vi "auto_alignment-v3-1.vi"(0 "meter-visa":refnum<visa-resource-name>, 1 "xStart":dbl=264.0 format="%#_13g", 2 "yStart":dbl=123.0 format="%#_13g", 3 "NM-params":T2={"alpha"=1.0, "gamma"=2.0, "rho"=0.5, "sigma"=0.5, "simplex L"=0.5}, 5 "PD Values":cluster{"PD1":dbl, "PD2":dbl, "PD3":dbl}, 7 "stage-refs":T1, 8 "NM-pts-tested":refnum<vi>, 9 "meter-error":errorcluster, 11 "stage-error":errorcluster, 12 "bar-note":u8, 13 "meas#":dbl format="%#_13g") -> (4 "Optimized Location":dbl[](array[numeric]), 6 "logfile-line-out":string, 10 "meter-error-out":errorcluster, 14 "run time (s)":dbl, 15 "stage-error-out":errorcluster)   [LabVIEW 2024]
uses:
  C:/Users/hpDIRC/Desktop/eic_dirc_daq-LabVIEW_new/Thorlabs.MotionControl.IntegratedStepperMotorsCLI.dll
  Thorlabs.MotionControl.IntegratedStepperMotorsCLI.dll
  C:/Users/hpDIRC/Desktop/eic_dirc_daq-LabVIEW_new/Thorlabs.MotionControl.Benchtop.StepperMotorCLI.dll
  Thorlabs.MotionControl.Benchtop.StepperMotorCLI.dll
  5b59031f-b1ff-41af-80a7-e72a33ebffa1.vi
  <vilib>/Analysis/baseanly.llb/Real Dot Product.vi
  <vilib>/Array/Sort 2D Array - Pop Stack.vi
  <vilib>/Array/Sort 2D Array - Push Stack.vi
  5b59031f-b1ff-41af-80a7-e72a33ebffa1.vi/269d4b3b-47f5-49e3-8884-44851e4dd9d5.vi
  5b59031f-b1ff-41af-80a7-e72a33ebffa1.vi/6d99389c-673d-4efb-bf33-19b32bcf4cf8.vi
  <vilib>/Analysis/NI_AALBase.lvlib
  <vilib>/Analysis/NI_AALPro.lvlib
panel:
  in  "fpga-ref-in":refnum<k20>
  out "z-angle converge":bool
  in  "z-angle-limit":dbl=0.04 caption="Z-Angle Convergence Goal"
  in  "squError-limit":dbl=0.04 caption="Squared Error Convergence Goal"
  out "angle-to-z":dbl
  out "squared error limit":bool
  out "SquError":dbl
  out "x_c":dbl[](array[numeric])
  out "x_e":dbl[](array[numeric])
  out "x_r":dbl[](array[numeric])
  out "x_o":dbl[](array[numeric])
  out "termination-test-simplex":dbl[][](array[numeric])
  out "timeout":bool
  out "simplex converge":bool
  out "value converge":bool
  out "simplex leg lengths":dbl[](array[numeric])
  out "std dev of simplex values":dbl
  out "nPts tested":dbl
  in  "simplex-limit":dbl=1e-06 caption="Simplex Length Convergence Goal" format="%#_13g"
  in  "value-limit":dbl=1e-06 caption="Value Convergence Goal" format="%#_13g"
  out "Pts Tested":dbl[][](array[numeric])
  in  "stop":bool
  # "Test Sub-Points"
  # "centroid"
  # "reflection point"
  # "expansion point"
  # "contraction point"
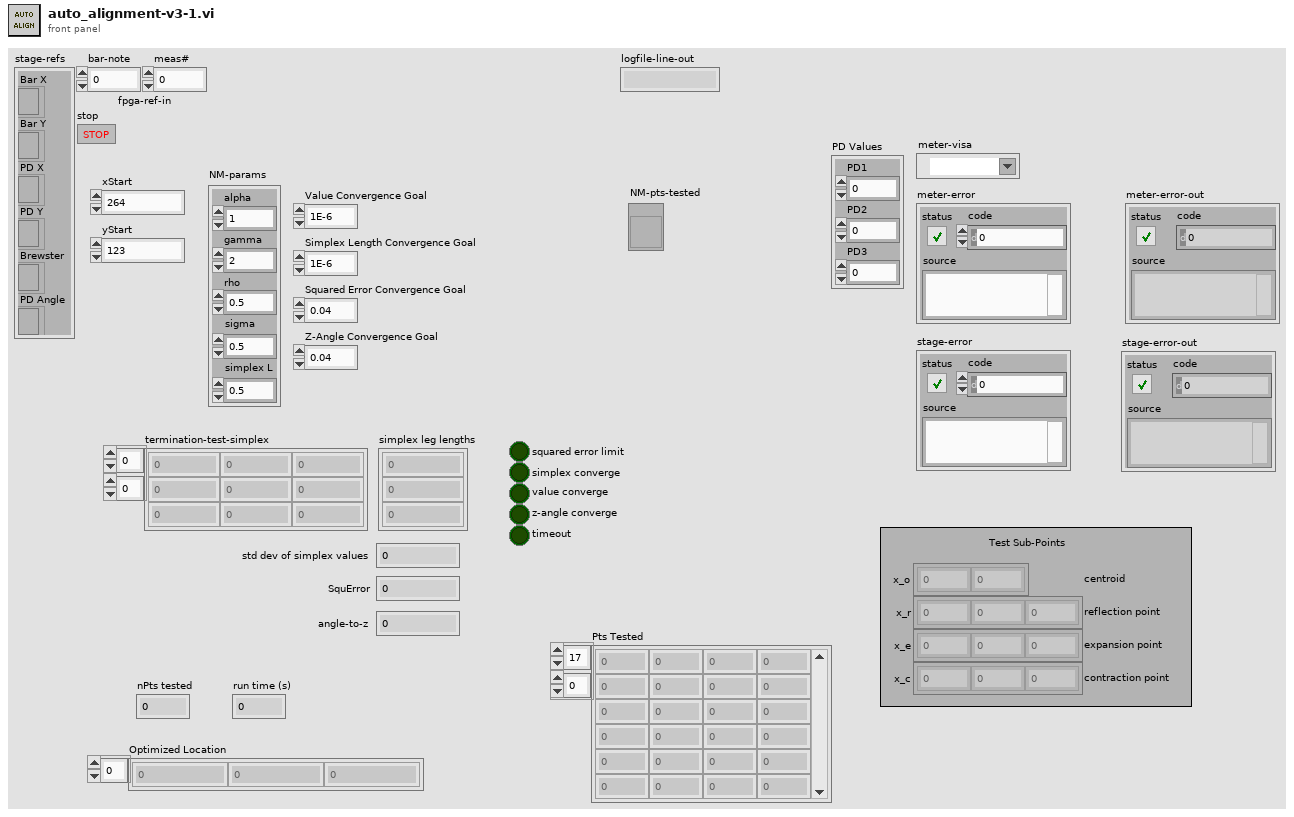
[diagram p1: front panel]
types:
  T1 = cluster{"Bar X":refnum<k24>, "Bar Y":refnum<k24>, "PD X":refnum<k24>, "PD Y":refnum<k24>, "Brewster":refnum<k24>, "PD Angle":refnum<k24>}
  T2 = cluster{"alpha":dbl, "gamma":dbl, "rho":dbl, "sigma":dbl, "simplex L":dbl}
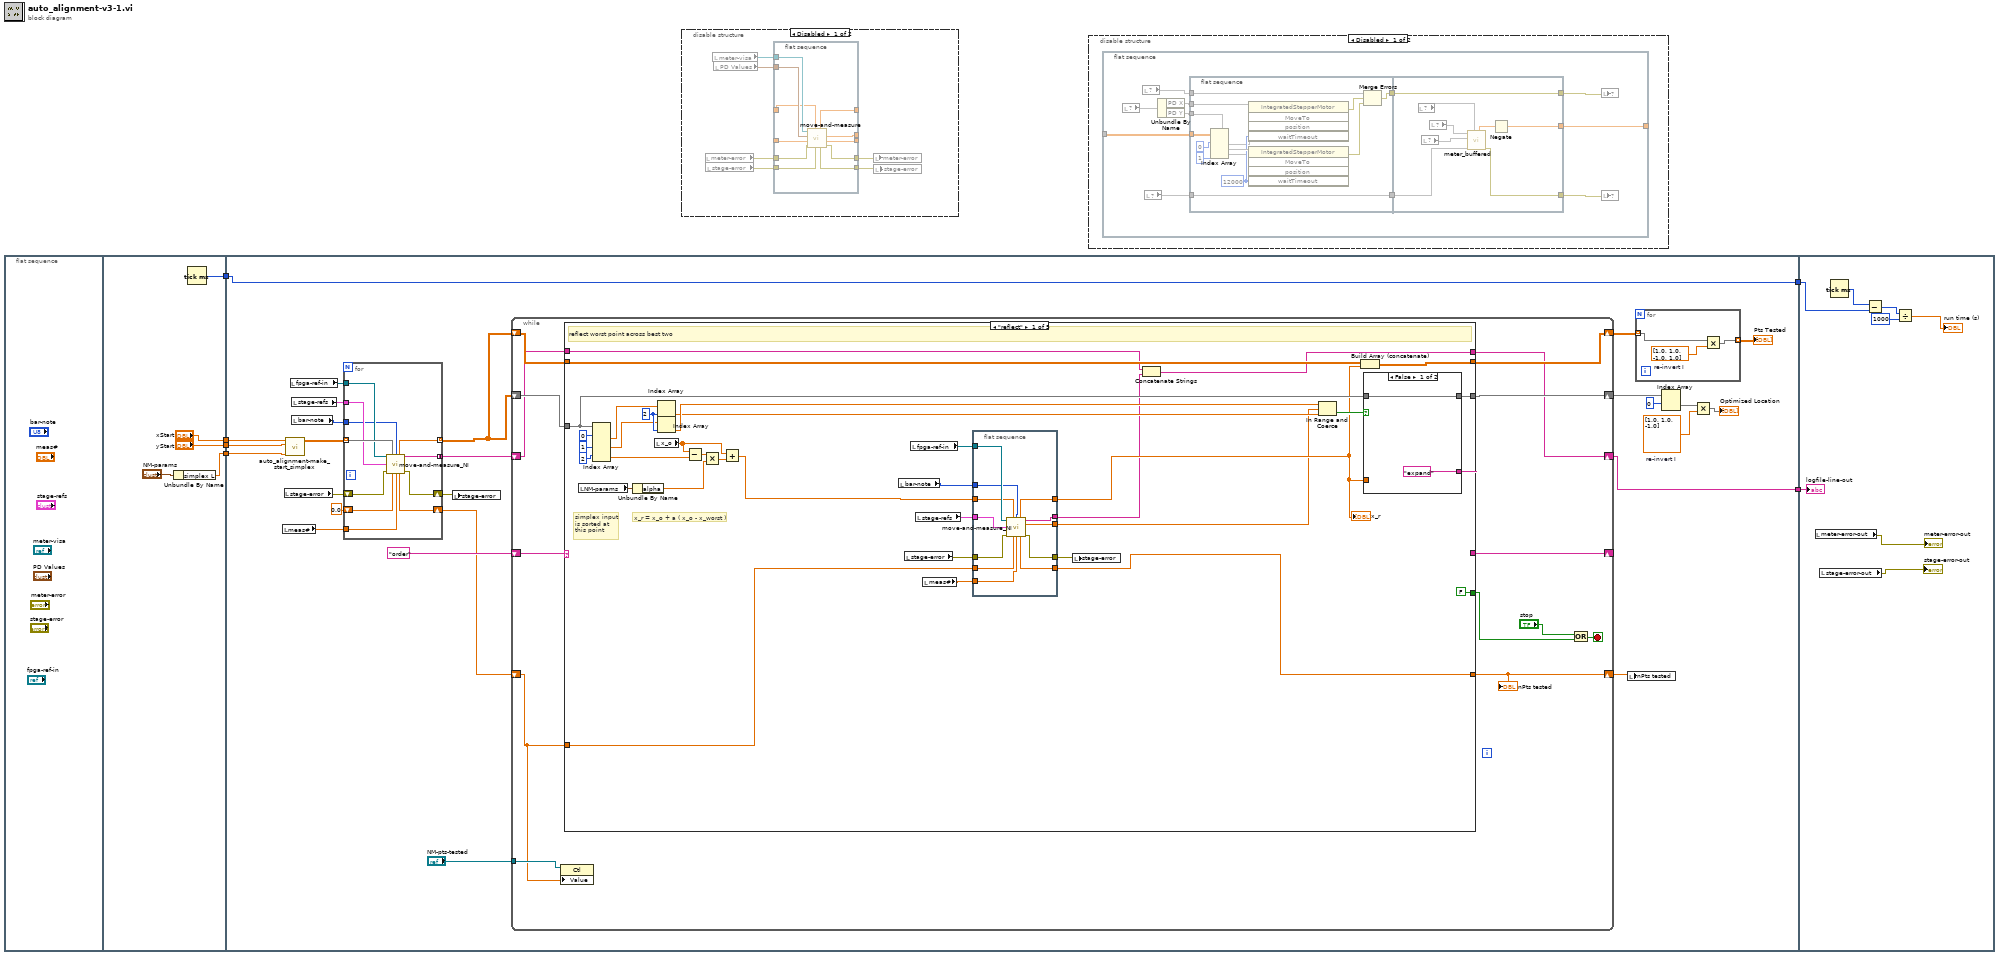
[diagram p0: block diagram]
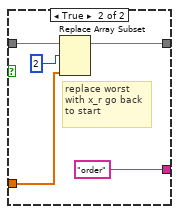
[diagram p4: hidden frame]
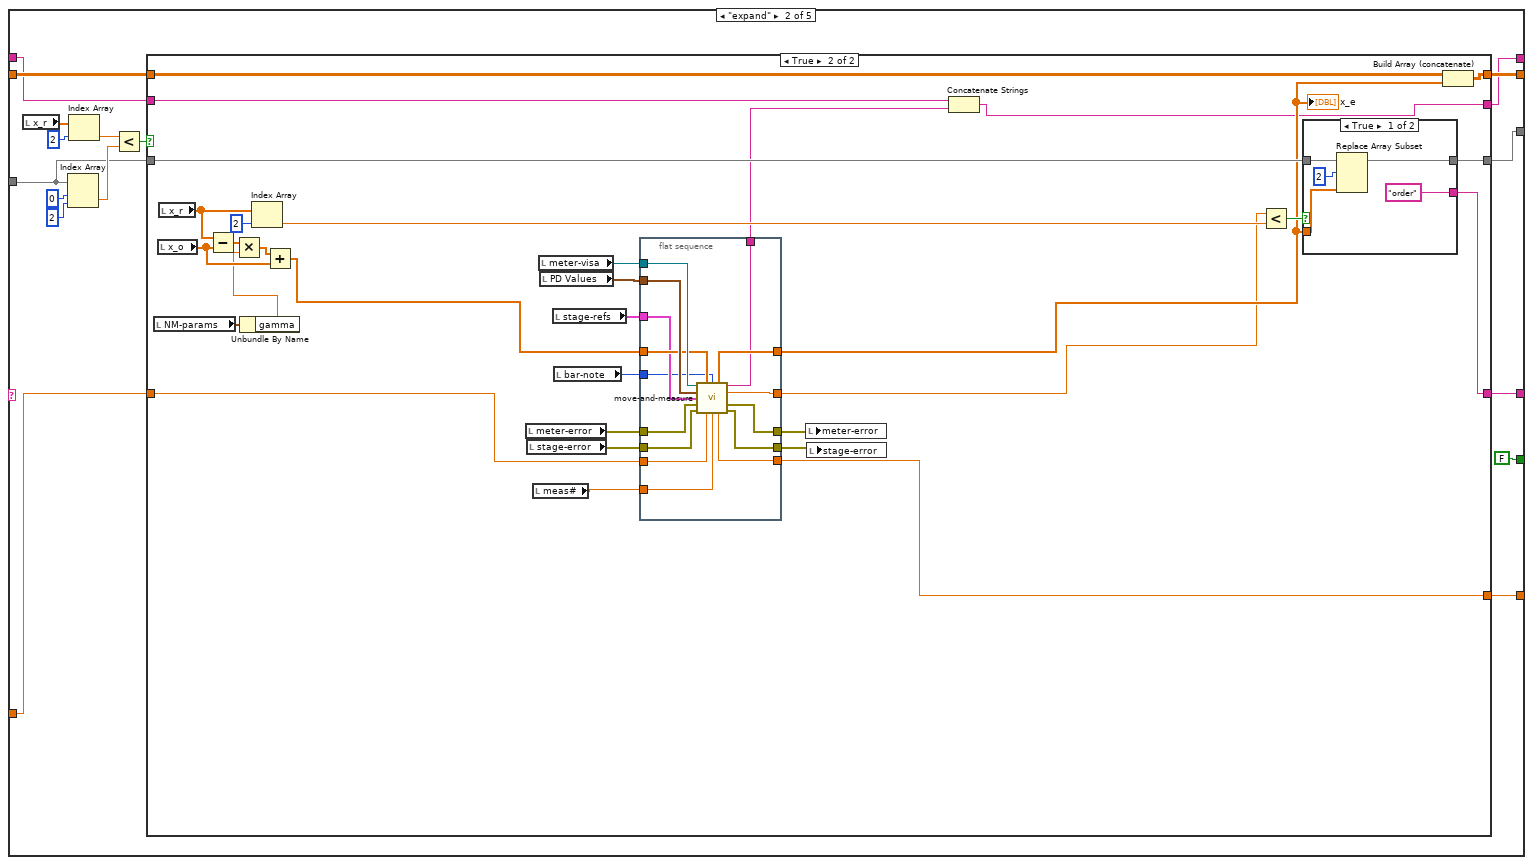
[diagram p5: hidden frame]
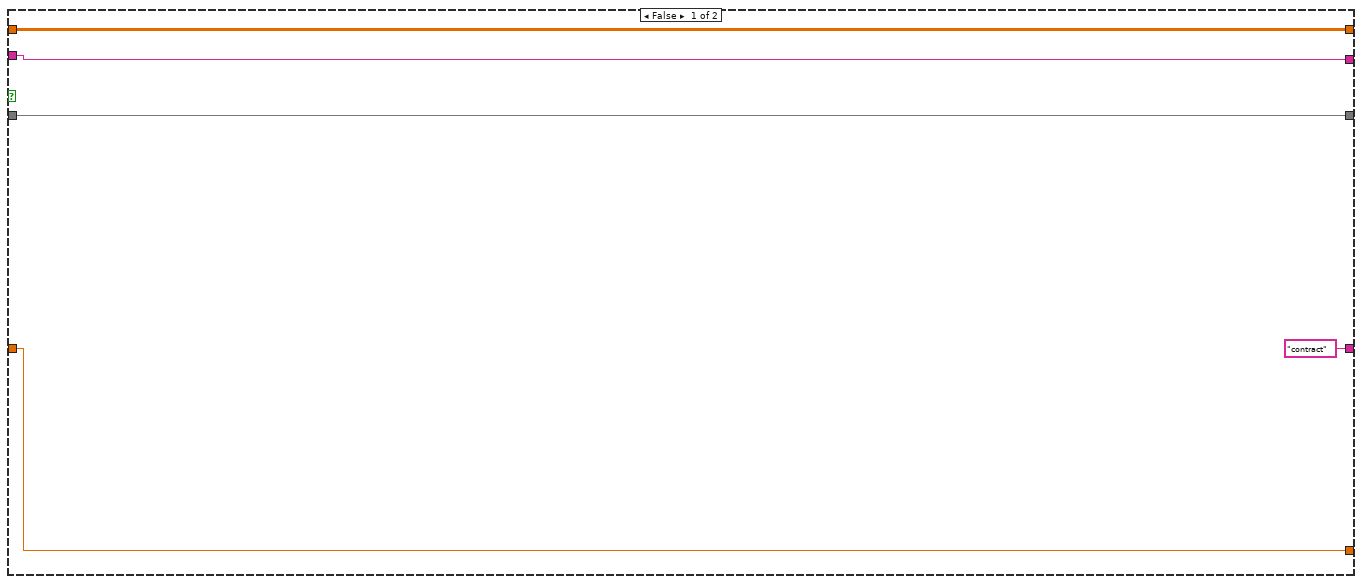
[diagram p6: hidden frame]
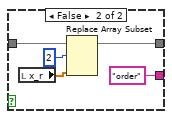
[diagram p7: hidden frame]
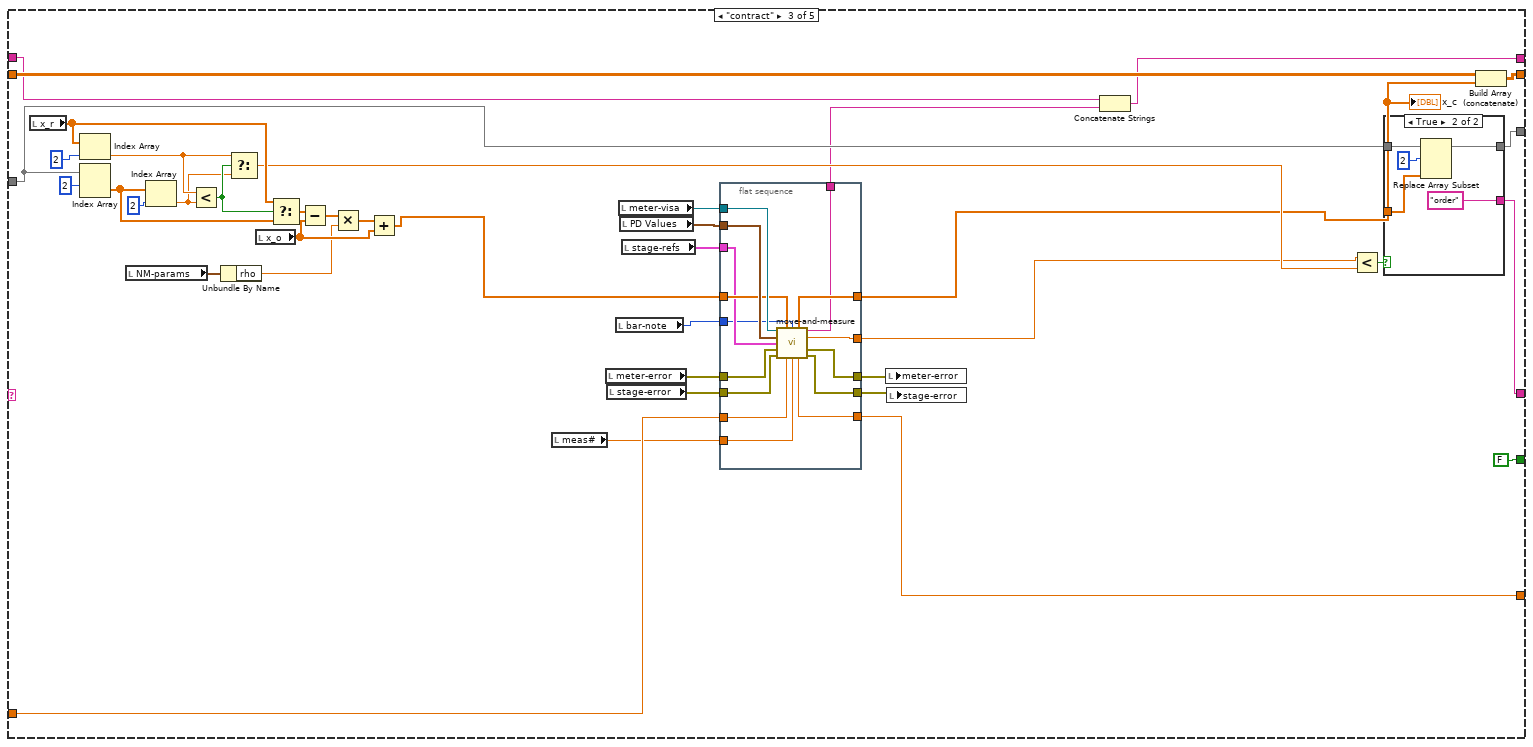
[diagram p8: hidden frame]
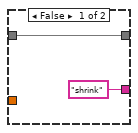
[diagram p9: hidden frame]
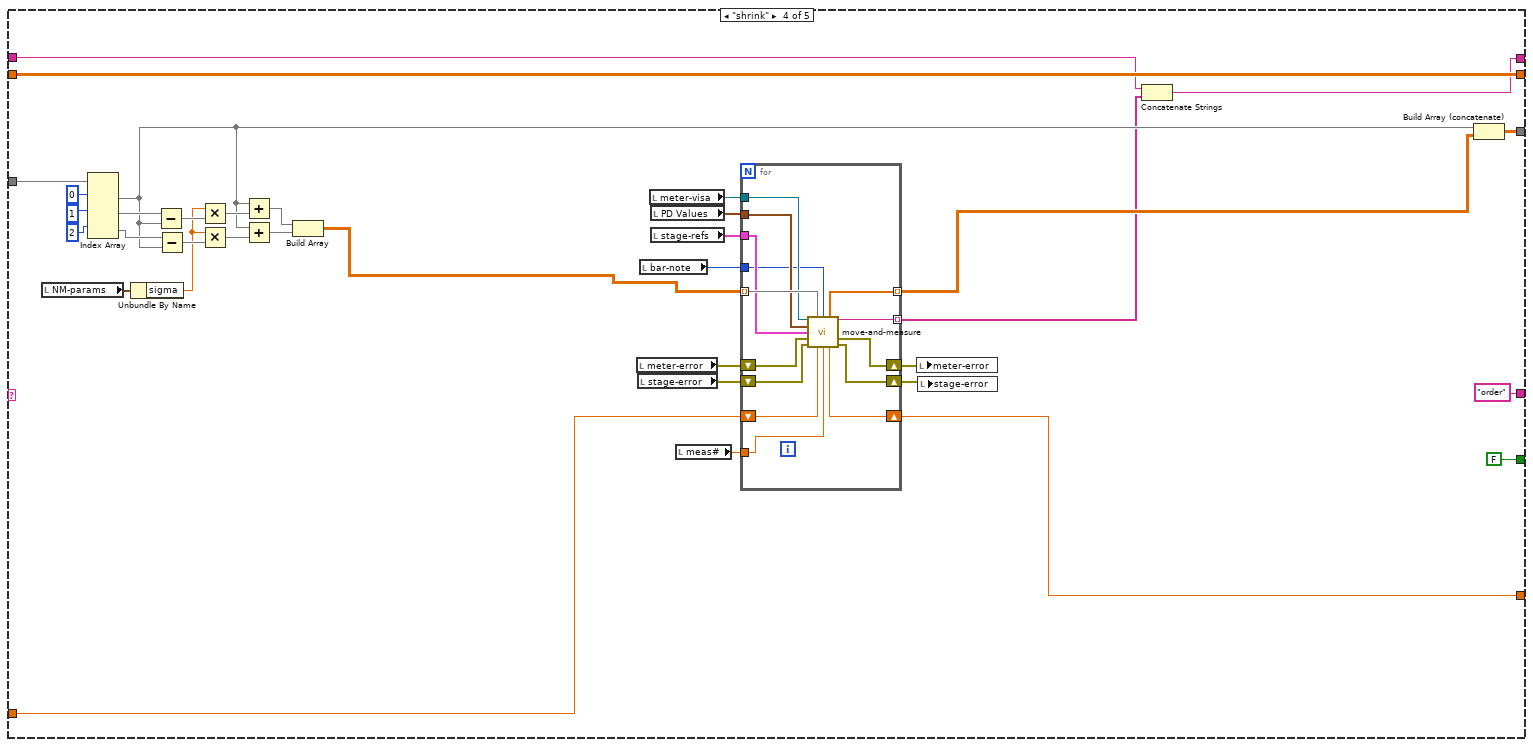
[diagram p10: hidden frame]
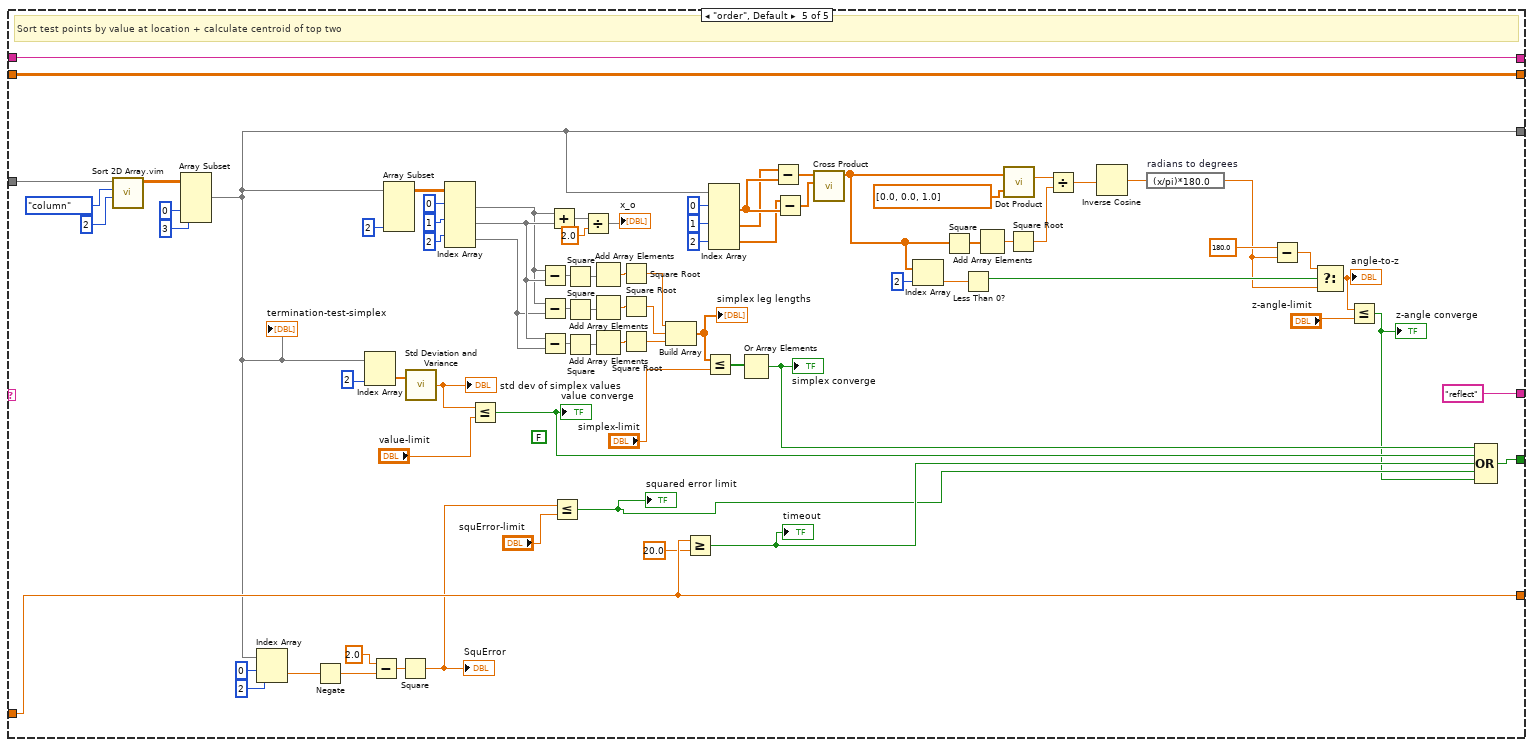
[diagram p11: hidden frame]
diagram:
  n1 = flat-sequence {
    tunnel: [w11] -> w6
    tunnel: ["yStart"] -> w4
    tunnel: ["xStart"] -> w3
    tunnel: [w9] -> w2
    tunnel: w6 -> [w36]
    tunnel: [w36] -> w5
    tunnel: w4 -> [w26]
    tunnel: w3 -> [w27]
    tunnel: w2 -> [w25]
    tunnel: [w15] -> w1
    tunnel: w5 -> [w394]
    tunnel: w1 -> [w388]
    frame #0 {
    }
    frame #1 {
      n2 = Unbundle By Name("NM-params") -> ("simplex L"=w9:dbl)
      n3 = Tick Count (ms)() -> (millisecond timer value=w11:u32)
    }
    frame #2 {
      w31 = dbl[] [1.0, 1.0, -1.0]  # re-invert I
      n4 = local read "meas#"() -> (w13:dbl)
      n5 = local read "stage-error"() -> (w19:errorcluster)
      n6 = call "auto_alignment-make_start_simplex.vi"("L"=w25, "yStart"=w26, "xStart"=w27) -> ("Array"=w28:dbl[][])  [unwired: 8 in]
      n7 = local read "fpga-ref-in"() -> (w30:refnum<k20>)
      n8 = local read "stage-refs"() -> (w17:T1)
      n9 = local read "bar-note"() -> (w14:u8)
      n10 = for {
        shift-right: [w44] -> w23
        shift-left: 0.0 -> [w45]
        tunnel: w28 -> [w51] mode=indexing
        tunnel: [w50] -> w24 mode=indexing
        tunnel: w30 -> [w49]
        shift-right: [w46] -> w18
        shift-left: w19 -> [w47]
        tunnel: w17 -> [w48]
        tunnel: [w43] -> w16 mode=concatenating
        tunnel: w14 -> [w42]
        tunnel: w13 -> [w41]
        n11 = call "move-and-measure_NI.vi"("fpga-ref-in"=w49, "XY-in"=w51, "bar-note"=w42, "stage-refs"=w48, "stage-error-in"=w47, "counter-in"=w45, "meas#"=w41) -> ("measured-point out"=w50:dbl[], "logfile-line-out"=w43:string, "counter-out"=w44:dbl, "stage-error-out"=w46:errorcluster)  [unwired: 4 in, 1 out]
      }
      n12 = local write "stage-error"(w18) -> ()
      n13 = while {
        shift-right: [w63] -> w35
        shift-left: w24 -> [w62]
        shift-right: [w64] -> _
        shift-left: "order" -> [w65]
        shift-right: [w60] -> w21
        shift-left: w24 -> [w61]
        shift-right: [w56] -> w22
        shift-left: w23 -> [w52]
        shift-right: [w54] -> w15
        shift-left: w16 -> [w55]
        tunnel: "NM-pts-tested" -> [w53]
        stop <- w57 stop-if-true
        n14 = property class="Ctl"(reference=w53, "Value"=w52) -> ()  [unwired: 1 in, 2 out]
        n15 = case shown="\"reflect\"" w65 {
          tunnel: w62 -> [w86 w129 w223 w292 w353]
          tunnel: [FALSE FALSE FALSE FALSE w360] -> w59
          tunnel: [w85 w128 w224 w281 w331] -> w63
          tunnel: [w87 w127 w225 "order" "reflect"] -> w64
          tunnel: w61 -> [w83 w125 w219 w279 w357]
          tunnel: [w82 w124 w218 w279 w357] -> w60
          tunnel: w52 -> [w76 w123 w204 w268 w351]
          tunnel: [w75 w122 w205 w267 w351] -> w56
          tunnel: w55 -> [w71 w120 w200 w262 w308]
          tunnel: [w70 w121 w202 w263 w308] -> w54
          frame "reflect" {
            w94 = 2 ("index")
            # "simplex input\nis sorted at\nthis point"
            # "x_r = x_o + a ( x_o - x_worst )"
            # "reflect worst point across best two"
            n16 = local read "NM-params"() -> (w81:T2)
            n17 = Index Array(array=w86, index (row) #1=0 ("index (row)"), index (row) #2=1 ("index (row)"), index (row) #3=2 ("index (row)")) -> (element #1=w93:dbl[], element #2=w92:dbl[], element #3=w95:dbl[])  [unwired: 3 in]
            n18 = Unbundle By Name(w81) -> ("alpha"=w80:dbl)
            n19 = local read "x_o"() -> (w88:dbl[])
            n20 = Index Array(array=w93, index=w94) -> (element=w90:dbl)
            n21 = Index Array(array=w92, index=w94) -> (element=w91:dbl)
            n22 = Subtract(x=w88, y=w95) -> (x-y=w99:dbl[])
            n23 = Multiply(x=w99, y=w80) -> (x*y=w98:dbl[])
            n24 = Add(x=w88, y=w98) -> (x+y=w73:dbl[])
            n25 = local read "bar-note"() -> (w68:u8)
            n26 = local read "stage-error"() -> (w78:errorcluster)
            n27 = local read "fpga-ref-in"() -> (w79:refnum<k20>)
            n28 = local read "stage-refs"() -> (w66:T1)
            n29 = local read "meas#"() -> (w67:dbl)
            n30 = flat-sequence {
              tunnel: [w112] -> w77
              tunnel: w78 -> [w111]
              tunnel: w76 -> [w110]
              tunnel: w79 -> [w109]
              tunnel: w73 -> [w108]
              tunnel: [w107] -> w74
              tunnel: [w106] -> w75
              tunnel: [w105] -> w72
              tunnel: [w104] -> w69
              tunnel: w68 -> [w103]
              tunnel: w67 -> [w102]
              tunnel: w66 -> [w101]
              frame #0 {
                n31 = call "move-and-measure_NI.vi"("fpga-ref-in"=w109, "XY-in"=w108, "bar-note"=w103, "stage-refs"=w101, "stage-error-in"=w111, "counter-in"=w110, "meas#"=w102) -> ("measured-point out"=w107:dbl[], "logfile-line-out"=w104:string, "iCorr-out"=w105:dbl, "counter-out"=w106:dbl, "stage-error-out"=w112:errorcluster)  [unwired: 4 in]
              }
            }
            n32 = local write "stage-error"(w77) -> ()
            n33 = Concatenate Strings(w71, w69) -> (w70:string)
            n34 = In Range and Coerce(upper limit=w91, x=w72, lower limit=w90) -> (In Range?=w89:bool)  [unwired: 1 out]
            n35 = Build Array (concatenate)(w83, w74) -> (w82:dbl[][])
            n36 = case shown="False" w89 {
              tunnel: ["expand" "order"] -> w87
              tunnel: w86 -> [w113 w119]
              tunnel: [w113 w116] -> w85
              tunnel: w74 -> [_ w117]
              frame False {
              }
              frame True {
                # "replace worst \nwith x_r go back\nto start"
                n37 = Replace Array Subset(array=w119, new element=w117, index (row)=2) -> (w116:dbl[][])  [unwired: 1 in]
              }
            }
            "x_r" <- w74
          }
          frame "expand" {
            n38 = local read "x_r"() -> (w134:dbl[])
            n39 = Index Array(array=w129, index (row)=0, index (col)=2 ("disabled index (col)")) -> (element=w132:dbl)
            n40 = Index Array(array=w134, index=2) -> (element=w131:dbl)
            n41 = Less?(x=w131, y=w132) -> (x < y?=w130:bool)
            n42 = case shown="True" w130 {
              tunnel: w129 -> [w141 w165]
              tunnel: [w141 w164] -> w128
              tunnel: ["contract" w163] -> w127
              tunnel: w125 -> [w139 w162]
              tunnel: [w139 w161] -> w124
              tunnel: w123 -> [w138 w150]
              tunnel: [w138 w149] -> w122
              tunnel: [w137 w146] -> w121
              tunnel: w120 -> [w137 w144]
              frame False {
              }
              frame True {
                n43 = local read "NM-params"() -> (w160:T2)
                n44 = local read "x_o"() -> (w170:dbl[])
                n45 = local read "x_r"() -> (w169:dbl[])
                n46 = Subtract(x=w169, y=w170) -> (x-y=w172:dbl[])
                n47 = Unbundle By Name(w160) -> ("gamma"=w159:dbl)
                n48 = Multiply(x=w172, y=w159) -> (x*y=w171:dbl[])
                n49 = Index Array(array=w169, index=2) -> (element=w167:dbl)
                n50 = Add(x=w171, y=w170) -> (x+y=w152:dbl[])
                n51 = local read "meter-error"() -> (w157:errorcluster)
                n52 = local read "stage-error"() -> (w155:errorcluster)
                n53 = local read "meas#"() -> (w142:dbl)
                n54 = local read "meter-visa"() -> (w156:refnum<visa-resource-name>)
                n55 = local read "PD Values"() -> (w158:cluster{"PD1":dbl, "PD2":dbl, "PD3":dbl})
                n56 = local read "stage-refs"() -> (w147:T1)
                n57 = local read "bar-note"() -> (w143:u8)
                n58 = flat-sequence {
                  tunnel: [w187] -> w153
                  tunnel: [w186] -> w154
                  tunnel: w155 -> [w185]
                  tunnel: w150 -> [w184]
                  tunnel: w156 -> [w183]
                  tunnel: w157 -> [w182]
                  tunnel: w158 -> [w181]
                  tunnel: w152 -> [w180]
                  tunnel: [w179] -> w151
                  tunnel: [w178] -> w149
                  tunnel: [w177] -> w148
                  tunnel: w147 -> [w176]
                  tunnel: [w175] -> w145
                  tunnel: w143 -> [w174]
                  tunnel: w142 -> [w173]
                  frame #0 {
                    n59 = call "move-and-measure.vi"("meter-visa"=w183, "XY-in"=w180, "bar-note"=w174, "PD Values"=w181, "stage-refs"=w176, "meter-error-in"=w182, "stage-error-in"=w185, "counter-in"=w184, "meas#"=w173) -> ("measured-point out"=w179:dbl[], "logfile-line-out"=w175:string, "iCorr-out"=w177:dbl, "meter-error-out"=w187:errorcluster, "counter-out"=w178:dbl, "stage-error-out"=w186:errorcluster)  [unwired: 1 in]
                  }
                }
                n60 = local write "meter-error"(w153) -> ()
                n61 = local write "stage-error"(w154) -> ()
                n62 = Concatenate Strings(w144, w145) -> (w146:string)
                n63 = Less?(x=w148, y=w167) -> (x < y?=w166:bool)
                n64 = case shown="True" w166 {
                  tunnel: w165 -> [w191 w196]
                  tunnel: w151 -> [w190 _]
                  tunnel: [w189 w195] -> w164
                  tunnel: ["order" "order"] -> w163
                  frame True {
                    n65 = Replace Array Subset(array=w191, new element=w190, index (row)=2) -> (w189:dbl[][])  [unwired: 1 in]
                  }
                  frame False {
                    n66 = local read "x_r"() -> (w193:dbl[])
                    n67 = Replace Array Subset(array=w196, new element=w193, index (row)=2) -> (w195:dbl[][])  [unwired: 1 in]
                  }
                }
                n68 = Build Array (concatenate)(w162, w151) -> (w161:dbl[][])
                "x_e" <- w151
              }
            }
          }
          frame "contract" {
            n69 = local read "x_r"() -> (w233:dbl[])
            n70 = Index Array(array=w233, index=2) -> (element=w228:dbl)
            n71 = Index Array(array=w223, index (row)=2) -> (element=w232:dbl[])  [unwired: 1 in]
            n72 = local read "NM-params"() -> (w217:T2)
            n73 = Index Array(array=w232, index=2) -> (element=w227:dbl)
            n74 = Less?(x=w228, y=w227) -> (x < y?=w229:bool)
            n75 = Unbundle By Name(w217) -> ("rho"=w216:dbl)
            n76 = Select(t=w228, s=w229, f=w227) -> (s? t:f=w215:dbl)
            n77 = local read "x_o"() -> (w221:dbl[])
            n78 = Select(t=w233, s=w229, f=w232) -> (s? t:f=w231:dbl[])
            n79 = Subtract(x=w231, y=w221) -> (x-y=w230:dbl[])
            n80 = Multiply(x=w230, y=w216) -> (x*y=w222:dbl[])
            n81 = Add(x=w222, y=w221) -> (x+y=w208:dbl[])
            n82 = local read "meas#"() -> (w198:dbl)
            n83 = local read "meter-error"() -> (w213:errorcluster)
            n84 = local read "stage-error"() -> (w211:errorcluster)
            n85 = local read "bar-note"() -> (w199:u8)
            n86 = local read "meter-visa"() -> (w212:refnum<visa-resource-name>)
            n87 = local read "PD Values"() -> (w214:cluster{"PD1":dbl, "PD2":dbl, "PD3":dbl})
            n88 = local read "stage-refs"() -> (w203:T1)
            n89 = flat-sequence {
              tunnel: [w251] -> w209
              tunnel: [w250] -> w210
              tunnel: w211 -> [w249]
              tunnel: w204 -> [w248]
              tunnel: w212 -> [w247]
              tunnel: w213 -> [w246]
              tunnel: w214 -> [w245]
              tunnel: w208 -> [w244]
              tunnel: [w243] -> w207
              tunnel: [w242] -> w205
              tunnel: [w241] -> w206
              tunnel: w203 -> [w240]
              tunnel: [w239] -> w201
              tunnel: w199 -> [w238]
              tunnel: w198 -> [w237]
              frame #0 {
                n90 = call "move-and-measure.vi"("meter-visa"=w247, "XY-in"=w244, "bar-note"=w238, "PD Values"=w245, "stage-refs"=w240, "meter-error-in"=w246, "stage-error-in"=w249, "counter-in"=w248, "meas#"=w237) -> ("measured-point out"=w243:dbl[], "logfile-line-out"=w239:string, "iCorr-out"=w241:dbl, "meter-error-out"=w251:errorcluster, "counter-out"=w242:dbl, "stage-error-out"=w250:errorcluster)  [unwired: 1 in]
              }
            }
            n91 = local write "meter-error"(w209) -> ()
            n92 = local write "stage-error"(w210) -> ()
            n93 = Concatenate Strings(w200, w201) -> (w202:string)
            n94 = Less?(x=w206, y=w215) -> (x < y?=w226:bool)
            n95 = case shown="True" w226 {
              tunnel: ["shrink" "order"] -> w225
              tunnel: [w252 w254] -> w224
              tunnel: w223 -> [w252 w256]
              tunnel: w207 -> [_ w255]
              frame False {
              }
              frame True {
                n96 = Replace Array Subset(array=w256, new element=w255, index (row)=2) -> (w254:dbl[][])  [unwired: 1 in]
              }
            }
            n97 = Build Array (concatenate)(w219, w207) -> (w218:dbl[][])
            "x_c" <- w207
          }
          frame "shrink" {
            n98 = local read "NM-params"() -> (w276:T2)
            n99 = Index Array(array=w292, index (row) #1=0 ("index (row)"), index (row) #2=1 ("index (row)"), index (row) #3=2 ("index (row)")) -> (element #1=w282:dbl[], element #2=w288:dbl[], element #3=w287:dbl[])  [unwired: 3 in]
            n100 = Unbundle By Name(w276) -> ("sigma"=w275:dbl)
            n101 = Subtract(x=w288, y=w282) -> (x-y=w285:dbl[])
            n102 = Subtract(x=w287, y=w282) -> (x-y=w286:dbl[])
            n103 = Multiply(x=w275, y=w285) -> (x*y=w284:dbl[])
            n104 = Multiply(x=w275, y=w286) -> (x*y=w283:dbl[])
            n105 = Add(x=w282, y=w284) -> (x+y=w278:dbl[])
            n106 = Add(x=w282, y=w283) -> (x+y=w277:dbl[])
            n107 = Build Array(w278, w277) -> (w265:dbl[][])
            n108 = local read "meter-error"() -> (w270:errorcluster)
            n109 = local read "stage-error"() -> (w272:errorcluster)
            n110 = local read "bar-note"() -> (w260:u8)
            n111 = local read "meter-visa"() -> (w271:refnum<visa-resource-name>)
            n112 = local read "PD Values"() -> (w269:cluster{"PD1":dbl, "PD2":dbl, "PD3":dbl})
            n113 = local read "stage-refs"() -> (w264:T1)
            n114 = local read "meas#"() -> (w259:dbl)
            n115 = for {
              shift-right: [w304] -> w267
              shift-left: w268 -> [w305]
              tunnel: w265 -> [w307] mode=indexing
              tunnel: [w306] -> w266 mode=indexing
              tunnel: w271 -> [w303]
              tunnel: w269 -> [w302]
              shift-right: [w299] -> w274
              shift-left: w270 -> [w301]
              shift-right: [w298] -> w273
              shift-left: w272 -> [w300]
              tunnel: w264 -> [w297]
              tunnel: [w296] -> w261 mode=indexing
              tunnel: w260 -> [w295]
              tunnel: w259 -> [w294]
              n116 = call "move-and-measure.vi"("meter-visa"=w303, "XY-in"=w307, "bar-note"=w295, "PD Values"=w302, "stage-refs"=w297, "meter-error-in"=w301, "stage-error-in"=w300, "counter-in"=w305, "meas#"=w294) -> ("measured-point out"=w306:dbl[], "logfile-line-out"=w296:string, "meter-error-out"=w299:errorcluster, "counter-out"=w304:dbl, "stage-error-out"=w298:errorcluster)  [unwired: 1 in, 1 out]
            }
            n117 = local write "meter-error"(w274) -> ()
            n118 = local write "stage-error"(w273) -> ()
            n119 = Concatenate Strings(w262, w261) -> (w263:string)
            n120 = Build Array (concatenate)(w282, w266) -> (w281:dbl[][])
          }
          frame "order", Default {
            (unwired) FALSE
            # "Sort test points by value at location + calculate centroid of top two"
            n121 = call "Sort 2D Array.vim"("index"=2, "dimension to index (column)"=enum16{"column", "row"}."column", "2D array"=w353) -> ("sorted 2D array"=w352:dbl[][])  [unwired: 7 in, 1 out]
            n122 = Array Subset(array=w352, index (col)=0 ("index"), length (col)=3 ("length")) -> (w331:dbl[][])  [unwired: 2 in]
            "termination-test-simplex" <- w331
            n123 = Index Array(array=w331, index (row)=0, index (col)=2 ("disabled index (col)")) -> (element=w346:dbl)
            n124 = Negate(x=w346) -> (-x=w344:dbl)
            n125 = Index Array(array=w331, index (col)=2 ("index")) -> (element=w377:dbl[])  [unwired: 1 in]
            n126 = Subtract(x=2.0, y=w344) -> (x-y=w345:dbl)
            n127 = Array Subset(array=w331, length (col)=2 ("length")) -> (w376:dbl[][])  [unwired: 3 in]
            n128 = Square(x=w345) -> (x^2=w343:dbl)
            "SquError" <- w343
            n129 = call <vilib>:"Std Deviation and Variance.vi"("X"=w377) -> ("standard deviation"=w358:dbl)  [unwired: 1 in, 2 out]
            "std dev of simplex values" <- w358
            n130 = Index Array(array=w376, index (row) #1=0 ("index (row)"), index (row) #2=1 ("index (row)"), index (row) #3=2 ("index (row)")) -> (element #1=w341:dbl[], element #2=w342:dbl[], element #3=w340:dbl[])  [unwired: 3 in]
            n131 = Less Or Equal?(x=w358, y="value-limit") -> (x <= y?=w315:bool)
            "value converge" <- w315
            n132 = Subtract(x=w341, y=w342) -> (x-y=w374:dbl[])
            n133 = Subtract(x=w341, y=w340) -> (x-y=w366:dbl[])
            n134 = Subtract(x=w342, y=w340) -> (x-y=w369:dbl[])
            n135 = Add(x=w341, y=w342) -> (x+y=w381:dbl[])
            n136 = Less Or Equal?(x=w343, y="squError-limit") -> (x <= y?=w310:bool)
            "squared error limit" <- w310
            n137 = Square(x=w374) -> (x^2=w373:dbl[])
            n138 = Square(x=w366) -> (x^2=w370:dbl[])
            n139 = Square(x=w369) -> (x^2=w368:dbl[])
            n140 = Divide(x=w381, y=2.0) -> (x/y=→"x_o":dbl[])
            n141 = Add Array Elements(numeric array=w373) -> (sum=w372:dbl)
            n142 = Add Array Elements(numeric array=w370) -> (sum=w371:dbl)
            n143 = Add Array Elements(numeric array=w368) -> (sum=w367:dbl)
            n144 = Square Root(x=w372) -> (sqrt(x)=w363:dbl)
            n145 = Square Root(x=w371) -> (sqrt(x)=w364:dbl)
            n146 = Square Root(x=w367) -> (sqrt(x)=w365:dbl)
            n147 = Build Array(w363, w364, w365) -> (w362:dbl[])
            "simplex leg lengths" <- w362
            n148 = Greater Or Equal?(x=w351, y=20.0) -> (x >= y?=w349:bool)
            "timeout" <- w349
            n149 = Less Or Equal?(x=w362, y="simplex-limit") -> (x <= y?=w361:bool[])
            n150 = Index Array(array=w331, index (row) #1=0 ("index (row)"), index (row) #2=1 ("index (row)"), index (row) #3=2 ("index (row)")) -> (element #1=w327:dbl[], element #2=w326:dbl[], element #3=w325:dbl[])  [unwired: 3 in]
            n151 = Or Array Elements(Boolean array=w361) -> (logical OR=w359:bool)
            "simplex converge" <- w359
            n152 = Subtract(x=w326, y=w327) -> (x-y=w339:dbl[])
            n153 = Subtract(x=w325, y=w327) -> (x-y=w338:dbl[])
            n154 = call <vilib>:"Cross Product.vi"("B Vector"=w338, "A Vector"=w339) -> ("Cross Product"=w323:dbl[])  [unwired: 8 in, 1 out]
            n155 = Index Array(array=w323, index=2) -> (element=w321:dbl)
            n156 = Square(x=w323) -> (x^2=w337:dbl[])
            n157 = Less Than 0?(x=w321) -> (x < 0?=w320:bool)
            n158 = Add Array Elements(numeric array=w337) -> (sum=w336:dbl)
            n159 = call-poly <vilib>:"Dot Product.vi"("Y Vector"=dbl[] [0.0, 0.0, 1.0], "X Vector"=w323) -> ("X * Y"=w334:dbl)  [unwired: 1 out]
            n160 = Square Root(x=w336) -> (sqrt(x)=w333:dbl)
            n161 = Divide(x=w334, y=w333) -> (x/y=w324:dbl)
            n162 = Inverse Cosine(1:w324) -> (0:w332:dbl)
            n163 = expression code="(x/pi)*180.0" "radians to degrees"(w332) -> (w317:dbl)
            n164 = Subtract(x=180.0, y=w317) -> (x-y=w319:dbl)
            n165 = Select(t=w319, s=w320, f=w317) -> (s? t:f=w316:dbl)
            "angle-to-z" <- w316
            n166 = Less Or Equal?(x=w316, y="z-angle-limit") -> (x <= y?=w309:bool)
            "z-angle converge" <- w309
            n167 = Compound Arithmetic op=OR(w359, w315, w349, w310, w309) -> (w360:bool)
          }
        }
        "nPts tested" <- w56
        n168 = Compound Arithmetic op=OR("stop", w59) -> (w57:bool)
      }
      n169 = local write "nPts tested"(w22) -> ()
      n170 = for {
        tunnel: [w39] -> w20 mode=indexing
        tunnel: w21 -> [w40] mode=indexing
        w38 = dbl[] [1.0, 1.0, -1.0, 1.0]  # re-invert I
        n171 = Multiply(x=w40, y=w38) -> (x*y=w39:dbl[])
      }
      "Pts Tested" <- w20
      n172 = Index Array(array=w35, index (row)=0) -> (element=w32:dbl[])  [unwired: 1 in]
      n173 = Multiply(x=w32, y=w31) -> (x*y=→"Optimized Location":dbl[])
    }
    frame #3 {
      n174 = local read "meter-error-out"() -> (→"meter-error-out":errorcluster)
      n175 = local read "stage-error-out"() -> (→"stage-error-out":errorcluster)
      n176 = Tick Count (ms)() -> (millisecond timer value=w395:u32)
      n177 = Subtract(x=w395, y=w394) -> (x-y=w393:u32)
      n178 = Divide(x=w393, y=u32 1000) -> (x/y=→"run time (s)":dbl)
      "logfile-line-out" <- w388
    }
  }
  n179 = disable-structure shown="Disabled" {
    frame Disabled {
      n180 = local read "meter-error"() -> (w397:errorcluster)
      n181 = local read "stage-error"() -> (w399:errorcluster)
      n182 = local read "meter-visa"() -> (w398:refnum<visa-resource-name>)
      n183 = local read "PD Values"() -> (w396:cluster{"PD1":dbl, "PD2":dbl, "PD3":dbl})
      n184 = flat-sequence {
        tunnel: [w414] -> w401
        tunnel: [w413] -> w400
        tunnel: w399 -> [w412]
        tunnel: _ -> [w411]
        tunnel: w398 -> [w410]
        tunnel: w397 -> [w409]
        tunnel: w396 -> [w408]
        tunnel: [w407] -> w403
        tunnel: [w406] -> w402
        tunnel: [w405] -> _
        tunnel: [w404] -> _
        frame #0 {
          n185 = call "move-and-measure.vi"("stage-error-in"=w412, "XY-in"=w407, "meter-error-in"=w409, "counter-in"=w411, "PD Values"=w408, "meter-visa"=w410) -> ("meter-error-out"=w414:errorcluster, "counter-out"=w405:dbl, "iCorr-out"=w404:dbl, "stage-error-out"=w413:errorcluster, "measured-point out"=w406:dbl[])  [unwired: 1 in]
        }
      }
      n186 = local write "meter-error"(w401) -> ()
      n187 = local write "stage-error"(w400) -> ()
    }
    frame Enabled {
    }
  }
  n188 = disable-structure shown="Disabled" {
    frame Disabled {
      n189 = flat-sequence {
        tunnel: [w423] -> _
        tunnel: [w415] -> _
        frame #0 {
          n190 = local read item#-1() -> (w419)
          n191 = local read item#-1() -> (w420)
          n192 = local read item#-1() -> (w418)
          n193 = Unbundle By Name(w419) -> ("PD X"=w425, "PD Y"=w424)
          n194 = flat-sequence {
            tunnel: w425 -> [w436]
            tunnel: w424 -> [w435]
            tunnel: w420 -> [w429]
            tunnel: [w427] -> w415
            tunnel: w418 -> [w426]
            tunnel: [w428] -> w417
            tunnel: [w426] -> w416
            tunnel: [w446] -> w421
            tunnel: [w443] -> w422
            tunnel: [w439] -> w423
            tunnel: w417 -> [w446]
            tunnel: w416 -> [w444]
            frame #0 {
              w434 = 12000 ("waitTimeout")
              n195 = Index Array(array=w427, index (row) #1=0 ("index"), index (row) #2=1 ("index")) -> (element #1=w431, element #2=w430)  [unwired: 2 in]
              n196 = invoke class="IntegratedStepperMotor" method="MoveTo"(reference=w436, "position"=w431, "waitTimeout"=w434) -> (error out=w438:errorcluster)  [unwired: 2 in, 4 out]
              n197 = invoke class="IntegratedStepperMotor" method="MoveTo"(reference=w435, "position"=w430, "waitTimeout"=w434) -> (error out=w437:errorcluster)  [unwired: 2 in, 4 out]
              n198 = Merge Errors(w429, w438, w437) -> (w428:errorcluster)
            }
            frame #1 {
              n199 = local read item#-1() -> (w442)
              n200 = local read item#-1() -> (w440)
              n201 = local read item#-1() -> (w441)
              n202 = call "meter_buffered.vi"("Samples"=w442, "error in"=w444, "PD ranges"=w440, "meter-VISA"=w441) -> ("error out"=w443:errorcluster, "iCorr"=w445:dbl)  [unwired: 3 in, 3 out]
              n203 = Negate(x=w445) -> (-x=w439:dbl)
            }
          }
          n204 = local write item#-1(w421) -> ()
          n205 = local write item#-1(w422) -> ()
        }
      }
    }
    frame Enabled {
    }
  }
